vi "axes_auto_range.vi"(8 "Acutal Range":T2={"X"={"Min"=inf, "Max"=-inf}, "Y"={"Min"=inf, "Max"=-inf}, "Z"={"Min"=inf, "Max"=-inf}, "Amplitude"={"Min"=0.0, "Max"=0.0}}, 9 "Auto Range On":T4, 10 "Set Range To":T2) -> (0 "Translate":T1, 1 "Scale":T1, 2 "Range Min/Max":T2)   [LabVIEW 2020, in "3DPC_SurfacePlot.xctl"]
uses:
  <vilib>/Native 3D Graph/xcontrol/3DPC_SurfacePlot.xctl
  <vilib>/Native 3D Graph/typedefs/range_cluster.ctl
  <vilib>/Native 3D Graph/typedefs/min_max.ctl
  <vilib>/Native 3D Graph/typedefs/prop_axes_autorange.ctl
  <vilib>/Native 3D Graph/typedefs/vector.ctl
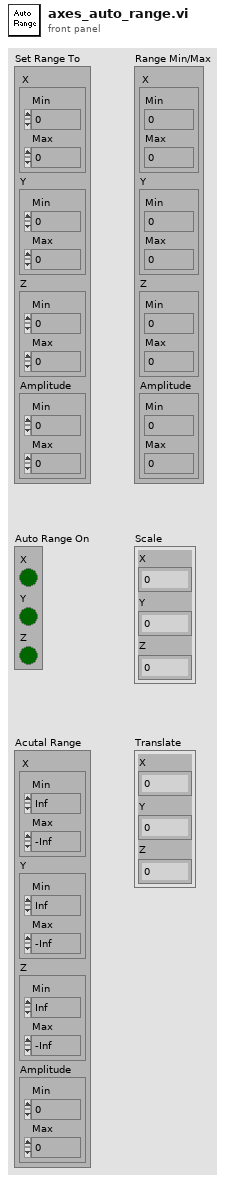
[diagram p1: front panel]
types:
  T1 = typedef "3DPC_SurfacePlot.xctl/vector.ctl" = cluster{"X":sgl, "Y":sgl, "Z":sgl}
  T2 = typedef "3DPC_SurfacePlot.xctl/range_cluster.ctl" = cluster{"X":T3, "Y":T3, "Z":T3, "Amplitude":T3}
  T3 = typedef "3DPC_SurfacePlot.xctl/min_max.ctl" = cluster{"Min":sgl, "Max":sgl}
  T4 = typedef "3DPC_SurfacePlot.xctl/prop_axes_autorange.ctl" = cluster{"X":bool, "Y":bool, "Z":bool}
  T5 = cluster{"Range":dbl, "Range 2":dbl, "Range 3":dbl}
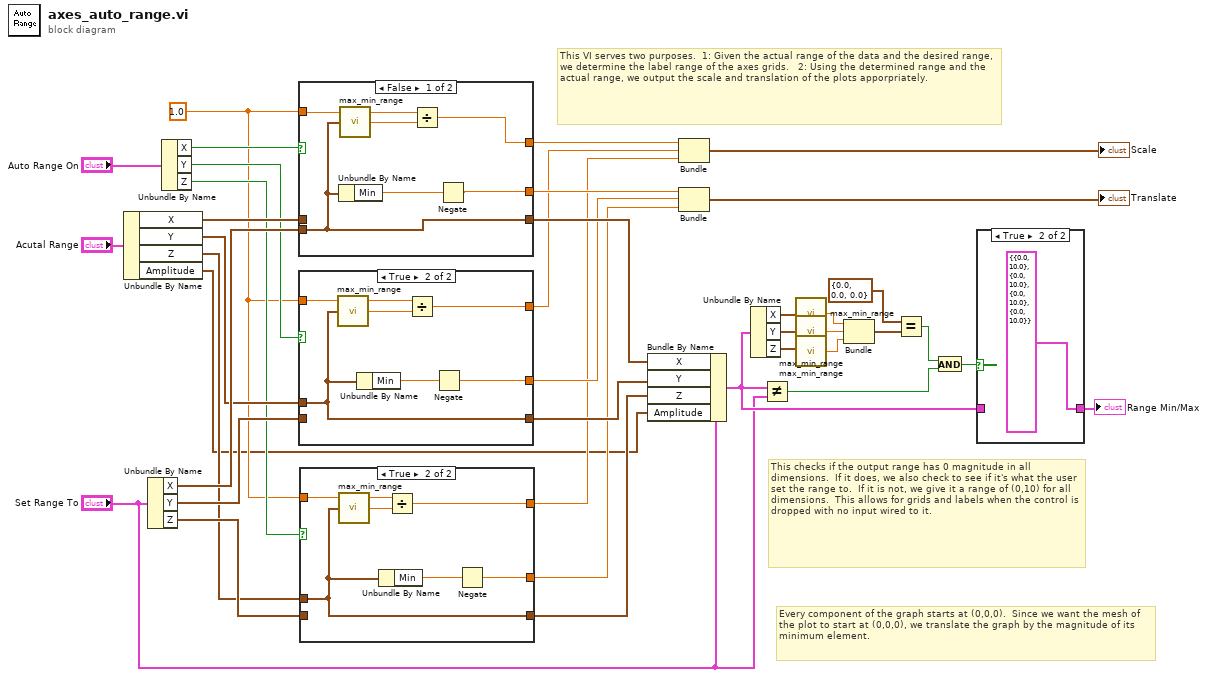
[diagram p0: block diagram]
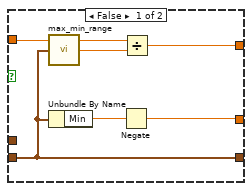
[diagram p2: hidden frame]
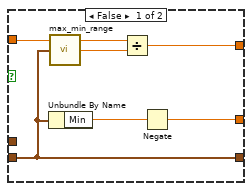
[diagram p3: hidden frame]
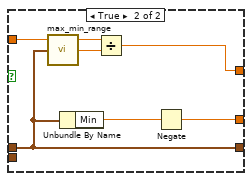
[diagram p4: hidden frame]
diagram:
  w16 = 1.0 ("Numeric")
  # "This checks if the output range has 0 magnitude in all dimensions.  If it does, we also check to see if it's what the user set the range to.  If it is not, we give it a range of (0,10) for all dimensions.  This allows for grids and labels when the control is dropped with no input wired to it."
  # "This VI serves two purposes.  1: Given the actual range of the data and the desired range, we determine the label range of the axes grids.   2: Using the determined range and the actual range, we output the scale and translation of the plots apporpriately."
  # "Every component of the graph starts at (0,0,0).  Since we want the mesh of the plot to start at (0,0,0), we translate the graph by the magnitude of its minimum element."
  n1 = Unbundle By Name("Acutal Range") -> ("X"=w35:T3, "Y"=w27:T3, "Z"=w17:T3, "Amplitude"=w1:T3)
  n2 = Unbundle By Name("Set Range To") -> ("X"=w34:T3, "Y"=w26:T3, "Z"=w18:T3)
  n3 = Unbundle By Name("Auto Range On") -> ("X"=w37:bool, "Y"=w28:bool, "Z"=w22:bool)
  n4 = case shown="False" w37 {
    tunnel: w35 -> [_ w45]
    tunnel: w34 -> [w42 _]
    tunnel: [w42 w45] -> w33
    tunnel: [w41 w48] -> w32
    tunnel: [w39 w46] -> w31
    tunnel: w16 -> [w44 w50]
    frame False {
      n5 = Unbundle By Name(w42) -> ("Min"=w40:sgl)
      n6 = call <vilib>:"max_min_range.vi"("Z Min/Max"=w42) -> ("Range"=w43:sgl)  [unwired: 8 out]
      n7 = Divide(x=w44, y=w43) -> (x/y=w41:dbl)
      n8 = Negate(x=w40) -> (-x=w39:sgl)
    }
    frame True {
      n9 = call <vilib>:"max_min_range.vi"("Z Min/Max"=w45) -> ("Range"=w49:sgl)  [unwired: 8 out]
      n10 = Unbundle By Name(w45) -> ("Min"=w47:sgl)
      n11 = Divide(x=w50, y=w49) -> (x/y=w48:dbl)
      n12 = Negate(x=w47) -> (-x=w46:sgl)
    }
  }
  n13 = case shown="True" w28 {
    tunnel: w27 -> [_ w58]
    tunnel: w26 -> [w54 _]
    tunnel: [w54 w58] -> w23
    tunnel: [w53 w60] -> w25
    tunnel: [w51 w57] -> w24
    tunnel: w16 -> [w56 w62]
    frame False {
      n14 = Unbundle By Name(w54) -> ("Min"=w52:sgl)
      n15 = call <vilib>:"max_min_range.vi"("Z Min/Max"=w54) -> ("Range"=w55:sgl)  [unwired: 8 out]
      n16 = Divide(x=w56, y=w55) -> (x/y=w53:dbl)
      n17 = Negate(x=w52) -> (-x=w51:sgl)
    }
    frame True {
      n18 = call <vilib>:"max_min_range.vi"("Z Min/Max"=w58) -> ("Range"=w61:sgl)  [unwired: 8 out]
      n19 = Unbundle By Name(w58) -> ("Min"=w59:sgl)
      n20 = Divide(x=w62, y=w61) -> (x/y=w60:dbl)
      n21 = Negate(x=w59) -> (-x=w57:sgl)
    }
  }
  n22 = case shown="True" w22 {
    tunnel: w17 -> [_ w71]
    tunnel: w18 -> [w66 _]
    tunnel: [w66 w71] -> w19
    tunnel: [w65 w72] -> w21
    tunnel: [w63 w69] -> w20
    tunnel: w16 -> [w68 w74]
    frame False {
      n23 = call <vilib>:"max_min_range.vi"("Z Min/Max"=w66) -> ("Range"=w67:sgl)  [unwired: 8 out]
      n24 = Unbundle By Name(w66) -> ("Min"=w64:sgl)
      n25 = Negate(x=w64) -> (-x=w63:sgl)
      n26 = Divide(x=w68, y=w67) -> (x/y=w65:dbl)
    }
    frame True {
      n27 = call <vilib>:"max_min_range.vi"("Z Min/Max"=w71) -> ("Range"=w73:sgl)  [unwired: 8 out]
      n28 = Unbundle By Name(w71) -> ("Min"=w70:sgl)
      n29 = Divide(x=w74, y=w73) -> (x/y=w72:dbl)
      n30 = Negate(x=w70) -> (-x=w69:sgl)
    }
  }
  n31 = Bundle By Name(cluster="Set Range To", "X"=w33, "Y"=w23, "Z"=w19, "Amplitude"=w1) -> (w4:T2)
  n32 = Bundle(w32, w25, w21) -> (→"Scale":cluster{dbl, dbl, dbl})  [unwired: 1 out]
  n33 = Bundle(w31, w24, w20) -> (→"Translate":cluster{sgl, sgl, sgl})  [unwired: 1 out]
  n34 = Unbundle By Name(w4) -> ("X"=w15:T3, "Y"=w14:T3, "Z"=w13:T3)
  n35 = Not Equal?(x=w4, y="Set Range To") -> (x != y?=w6:bool)
  n36 = call <vilib>:"max_min_range.vi"("Z Min/Max"=w15) -> ("Range"=w12:sgl)  [unwired: 8 out]
  n37 = call <vilib>:"max_min_range.vi"("Z Min/Max"=w14) -> ("Range"=w11:sgl)  [unwired: 8 out]
  n38 = call <vilib>:"max_min_range.vi"("Z Min/Max"=w13) -> ("Range"=w10:sgl)  [unwired: 8 out]
  n39 = Bundle("Range"=w12, "Range"=w11, "Range"=w10) -> (w9:cluster{"Range":sgl, "Range":sgl, "Range":sgl})  [unwired: 1 out]
  n40 = Equal?(x=T5 {"Range"=0.0, "Range 2"=0.0, "Range 3"=0.0}, y=w9) -> (x = y?=w7:bool)
  n41 = And(x=w7, y=w6) -> (x .and. y?=w5:bool)
  n42 = case shown="True" w5 {
    tunnel: w4 -> [w75 _]
    tunnel: [w75 T2 {"X"={"Min"=0.0, "Max"=10.0}, "Y"={"Min"=0.0, "Max"=10.0}, "Z"={"Min"=0.0, "Max"=10.0}, "Amplitude"={"Min"=0.0, "Max"=10.0}} ("Set Range To")] -> w3
    frame False {
    }
    frame True {
    }
  }
  "Range Min/Max" <- w3
